vi "Decode Parameters for Labels in a Channel.vi"(6 "labels settings for RT":T1[](array[typedef]) {"Label Timestamp Channel Data Reference" format="%.0x"; "Word Initial Raw Value" format="%032.0f"; "Label Disable/Trigger Channel Reference" format="%.0x"; "parameter driver data"."Tx parameter refs" format="%.0x"; "SDI" format="%02b"; "label" format="%.0o"}, 7 "reset index":bool, 8 "error in (no error)":errorcluster, 9 "updated labels?":bool[](array[boolean]), 10 "data words in":u32[](array[numeric]), 11 "Parameter Values in":dbl[](array[numeric])) -> (0 "error out":errorcluster, 3 "Parameter Values out":dbl[](array[numeric]))   [LabVIEW 2024, in "AIM ARINC 429 Engine.lvlib" / "Implementation.lvlib" / "Rx Execution Unit.lvclass"]
doc: "Decodes the parameters defined in parameter definitions section of a label settings cluster. Receives an array of data words (one per label in the channel), and an array of label settings (one per label in the channel). \n\nThis VI requires a preallocated array with a size equal to the number of parameters in all channels, and it will continue to replace items in the array, incrementing until a True is passed to reset index."
uses:
  Rx Execution Unit.lvclass
  Shared/RT Label Settings.ctl
  Shared/Label.ctl
  Shared/RT Parameters.ctl
  Shared/Parameter Definition.ctl
  <vilib>/NI/NI VeriStand Encoding and Decoding/Encoding.ctl
  <vilib>/NI VeriStand/Custom Device API/Custom Device Item Ref.ctl
  Shared/Transfer Type.ctl
  <vilib>/NI VeriStand/Custom Device API/Data Reference.ctl
  Shared/Decode Parameter (DBL) from Word.vi/1980749b-e417-4a21-943a-7c30016504b0.vi
  Shared/Decode Parameter (DBL) from Word.vi/1f3c3557-5c17-491c-9e18-ef0b55369bc3.vi
  Shared/Decode Parameter (DBL) from Word.vi/1980749b-e417-4a21-943a-7c30016504b0.vi/16a2565b-3c16-407b-a626-9da2a3da432e.vi
  Shared/Decode Parameter (DBL) from Word.vi/1f3c3557-5c17-491c-9e18-ef0b55369bc3.vi/0a001d06-2809-4638-8d0b-e017d2157007.vi
  Shared/Decode Parameter (DBL) from Word.vi/1f3c3557-5c17-491c-9e18-ef0b55369bc3.vi/e08d08e5-79bf-42ec-a5e5-c4db927cd1a5.vi
  <vilib>/NI/NI VeriStand Encoding and Decoding/Get Bits Per Digit from Base.vi
  <vilib>/NI/NI VeriStand Encoding and Decoding/Encoding and Decoding.lvlib
  <vilib>/NI VeriStand/Custom Device API/Custom Device API.lvlib
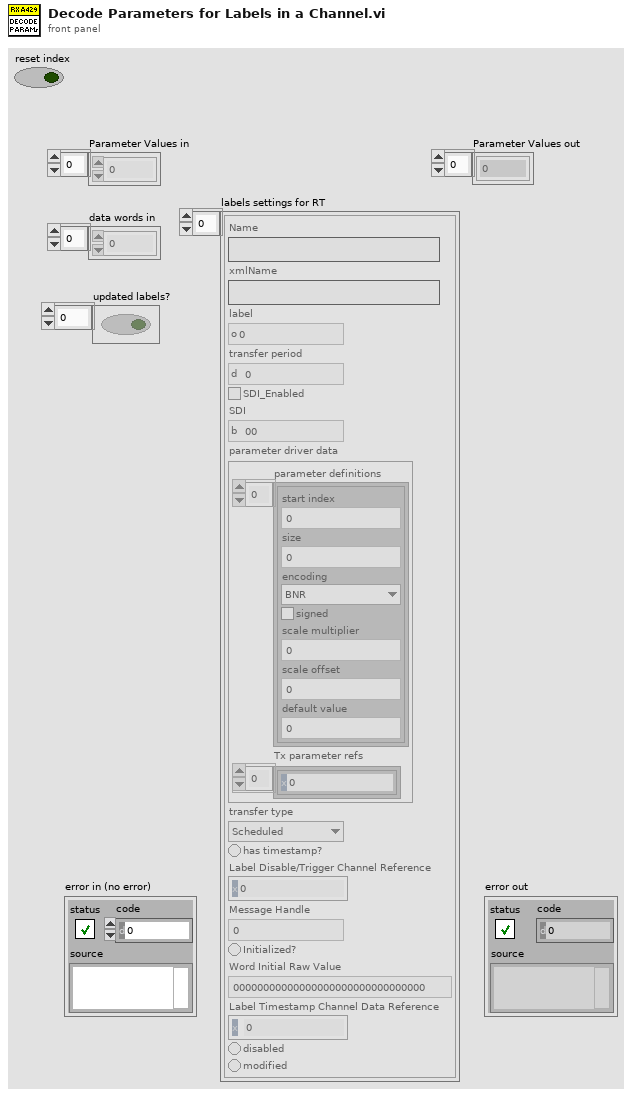
[diagram p1: front panel]
types:
  T1 = typedef "RT Label Settings.ctl" = cluster{"Name":string, "xmlName":string, "label":T2, "transfer period":u32, "SDI_Enabled":bool, "SDI":u8, "parameter driver data":T3, "transfer type":T7, "has timestamp?":bool, "Label Disable/Trigger Channel Reference":T6, "Message Handle":u64, "Initialized?":bool, "Word Initial Raw Value":u32, "Label Timestamp Channel Data Reference":T8, "disabled":bool, "modified":bool}
  T2 = typedef "Label.ctl" = u8
  T3 = typedef "RT Parameters.ctl" = cluster{"parameter definitions":T4[], "Tx parameter refs":T6[]}
  T4 = typedef "Parameter Definition.ctl" = cluster{"start index":i32, "size":i32, "encoding":T5, "signed":bool, "scale multiplier":dbl, "scale offset":dbl, "default value":dbl}
  T5 = typedef "Encoding and Decoding.lvlib/Encoding.ctl" = enum16{"BNR", "BCD", "Discrete"}
  T6 = typedef "Custom Device API.lvlib/Custom Device Item Ref.ctl" = u64
  T7 = typedef "Transfer Type.ctl" = enum16{"Scheduled", "Acyclic", "Block", "Strobe"}
  T8 = typedef "Custom Device API.lvlib/Data Reference.ctl" = i32
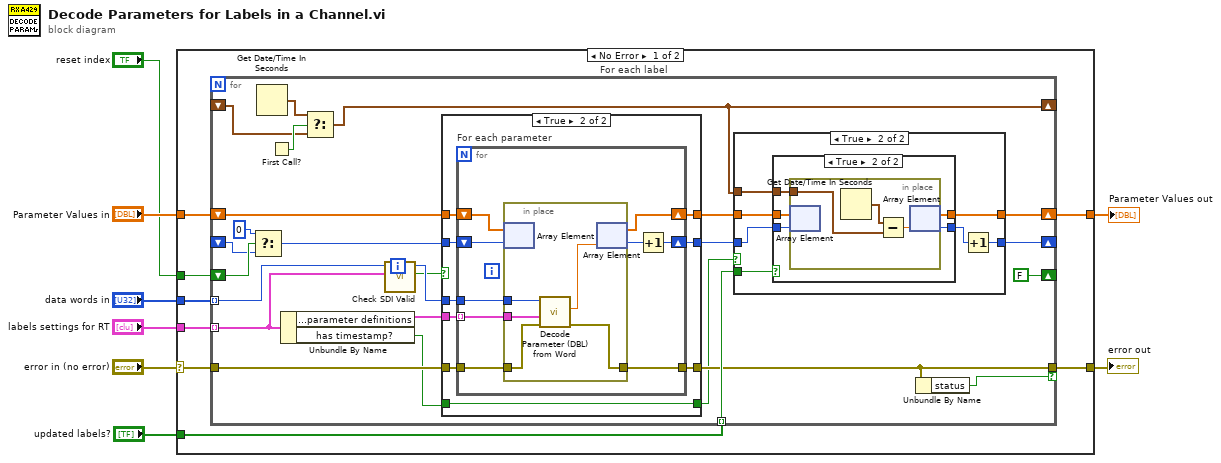
[diagram p0: block diagram]
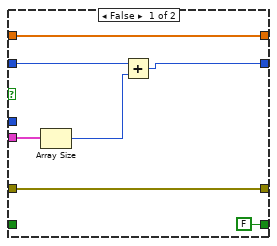
[diagram p2: hidden frame]
diagram:
  n1 = case shown="No Error" "error in (no error)" {
    selector: "error in (no error)" -> [w10 w92]
    tunnel: "data words in" -> [w16 _]
    tunnel: "labels settings for RT" -> [w15 _]
    tunnel: [w14 w92] -> w6
    tunnel: "Parameter Values in" -> [w13 w91]
    tunnel: [w12 w91] -> w4
    tunnel: "reset index" -> [w11 _]
    tunnel: "updated labels?" -> [w9 _]
    frame No Error {
      n2 = for "For each label" {
        tunnel: w16 -> [w22] mode=indexing
        tunnel: w15 -> [w20] mode=indexing
        shift-right: [w28] -> w12
        shift-left: w13 -> [w32]
        shift-right: [FALSE ("reset index")] -> _
        shift-left: w11 -> [w39]
        shift-right: [w29] -> _
        shift-left: _ -> [w37]
        tunnel: w9 -> [w36] mode=indexing
        shift-right: [w33] -> _
        shift-left: _ -> [w34]
        tunnel: w10 -> [w40]
        tunnel: [w24] -> w14 if=w23
        n3 = Select(t=0, s=w39, f=w37) -> (s? t:f=w31:i32)
        n4 = Get Date/Time In Seconds() -> (seconds since 1Jan1904=w25:timestamp)
        n5 = First Call?() -> (First Call?: T/F=w35:bool)
        n6 = Unbundle By Name(w20) -> ("parameter driver data.parameter definitions"=w41:T4[], "has timestamp?"=w18:bool)
        n7 = Select(t=w25, s=w35, f=w34) -> (s? t:f=w33:timestamp)
        n8 = call "Check SDI Valid.vi"("label settings for RT"=w20, "data word in"=w22) -> ("sdi valid?"=w19:bool, "data word out"=w21:u32)  [unwired: 8 in]
        n9 = case shown="True" w19 {
          tunnel: w41 -> [w43 w57]
          tunnel: w40 -> [w47 w56]
          tunnel: w32 -> [w48 w55]
          tunnel: w31 -> [w45 w54]
          tunnel: [w44 w53] -> w30
          tunnel: [w48 w52] -> w27
          tunnel: [w47 w51] -> w24
          tunnel: w21 -> [_ w50]
          tunnel: w18 -> [_ w49]
          tunnel: [FALSE ("has timestamp?") w49] -> w17
          frame False {
            n10 = Array Size(array=w43) -> (size(s)=w42:i32)
            n11 = Add(x=w45, y=w42) -> (x+y=w44:i32)
          }
          frame True {
            n12 = for "For each parameter" {
              tunnel: w50 -> [w66]
              tunnel: w57 -> [w65] mode=indexing
              shift-right: [w60] -> w52
              shift-left: w55 -> [w62]
              tunnel: w56 -> [w64]
              tunnel: [w63] -> w51
              shift-right: [w59] -> w53
              shift-left: w54 -> [w58]
              n13 = in-place {
                in-place-border: w66 -> [w71]
                in-place-border: w65 -> [w70]
                in-place-border: w64 -> [w69]
                in-place-border: [w68] -> w63
                n14 = in-place-array #1(w62, w58) -> ()  [unwired: 1 out]
                n15 = call "Decode Parameter (DBL) from Word.vi"("error in"=w69, "parameter definition"=w70, "32-bit word in"=w71) -> ("error out"=w68:errorcluster, "parameter value"=w67:dbl)  [unwired: 6 in, 1 out]
                n16 = in-place-array #1(w67) -> (w60:dbl[], w61:i32)
              }
              n17 = Increment(x=w61) -> (x+1=w59:i32)
            }
          }
        }
        n18 = case shown="True" w17 {
          tunnel: w30 -> [w73 w79]
          tunnel: [w73 w78] -> w29
          tunnel: w27 -> [w72 w80]
          tunnel: [w72 w76] -> w28
          tunnel: w36 -> [_ w75]
          tunnel: w33 -> [_ w74]
          frame False {
          }
          frame True {
            n19 = case shown="True" w75 {
              tunnel: w80 -> [w82 w87]
              tunnel: w79 -> [w81 w86]
              tunnel: [w81 w85] -> w77
              tunnel: [w82 w84] -> w76
              tunnel: w74 -> [_ w83]
              frame False {
              }
              frame True {
                n20 = in-place {
                  in-place-border: w83 -> [w89]
                  n21 = in-place-array #2(w87, w86) -> ()  [unwired: 1 out]
                  n22 = Get Date/Time In Seconds() -> (seconds since 1Jan1904=w90:timestamp)
                  n23 = Subtract(x=w90, y=w89) -> (x-y=w88:dbl)
                  n24 = in-place-array #2(w88) -> (w84:dbl[], w85:i32)
                }
              }
            }
            n25 = Increment(x=w77) -> (x+1=w78:i32)
          }
        }
        n26 = Unbundle By Name(w24) -> ("status"=w23:bool)
      }
    }
    frame Error {
    }
  }
  "error out" <- w6
  "Parameter Values out" <- w4
